vi "GOOP_ArrayInsert.vi"(0 "ArrayIn":string[][](array[string]), 1 "Text":string, 2 "Row":i32, 3 "Column":i32) -> (14 "ArrayOut":string[][](array[string]))   [LabVIEW 2020]
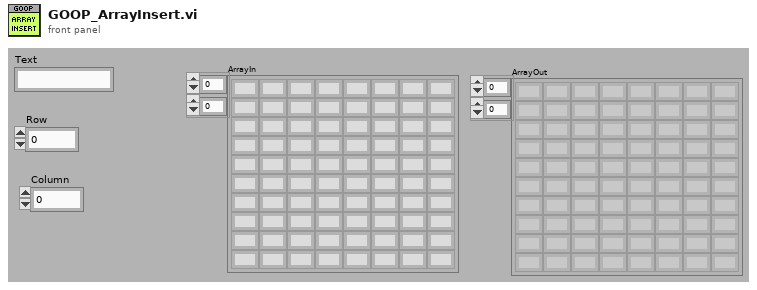
[diagram p1: front panel]
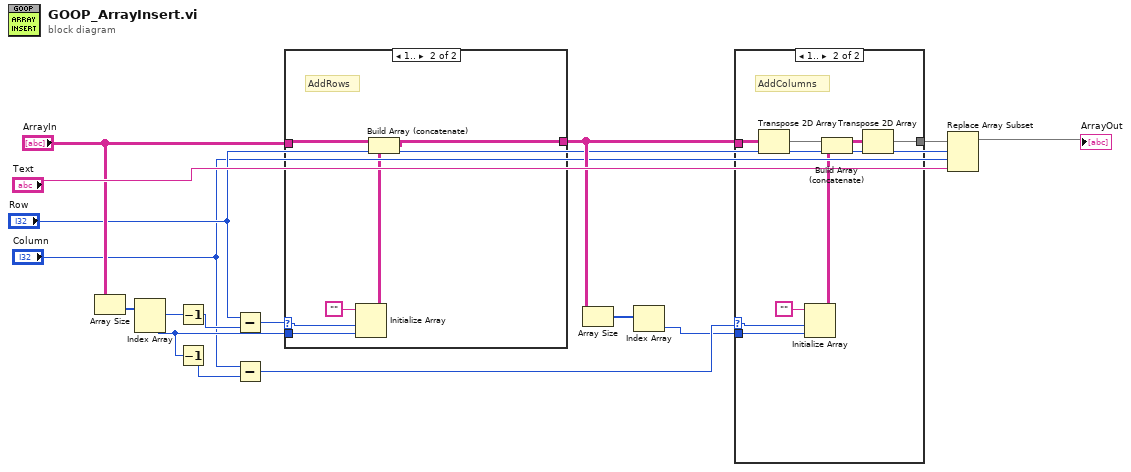
[diagram p0: block diagram]
diagram:
  n1 = Array Size(array="ArrayIn") -> (size(s)=w12:i32[])
  n2 = Index Array(array=w12) -> (element #1=w11:i32, element #2=w9:i32)  [unwired: 2 in]
  n3 = Decrement(x=w11) -> (x-1=w10:i32)
  n4 = Decrement(x=w9) -> (x-1=w8:i32)
  n5 = Subtract(x="Row", y=w10) -> (x-y=w14:i32)
  n6 = Subtract(x="Column", y=w8) -> (x-y=w7:i32)
  n7 = case shown="1.." w14 {
    selector: w14 -> [_ w21]
    tunnel: "ArrayIn" -> [w17 w19]
    tunnel: [w17 w18] -> w6
    tunnel: w9 -> [_ w20]
    frame 0, Default {
    }
    frame 1.. {
      # "AddRows"
      n8 = Initialize Array("", w21, w20) -> (w23:string[][])
      n9 = Build Array (concatenate)(w19, w23) -> (w18:string[][])
    }
  }
  n10 = Array Size(array=w6) -> (size(s)=w5:i32[])
  n11 = Index Array(array=w5) -> (element=w4:i32)  [unwired: 1 in]
  n12 = case shown="1.." w7 {
    selector: w7 -> [_ w28]
    tunnel: w6 -> [w24 w32]
    tunnel: [w24 w25] -> w3
    tunnel: w4 -> [_ w27]
    frame 0, Default {
    }
    frame 1.. {
      # "AddColumns"
      n13 = Transpose 2D Array(2D array=w32) -> (transposed array=w26:string[][])
      n14 = Initialize Array("", w28, w27) -> (w30:string[][])
      n15 = Build Array (concatenate)(w26, w30) -> (w31:string[][])
      n16 = Transpose 2D Array(2D array=w31) -> (transposed array=w25:string[][])
    }
  }
  n17 = Replace Array Subset(array=w3, new element="Text", index (row)="Row", index (col)="Column") -> (→"ArrayOut":string[][])
